vi "test Script Bitfile.vi"(8 "error in (no error)":errorcluster, 11 "TestCase in":refnum<class "Scripting API Test Case.lvclass">) -> (0 "error out":errorcluster, 3 "TestCase out":refnum<class "Scripting API Test Case.lvclass">)   [LabVIEW 2015, in "Scripting API Test Case.lvclass"]
uses:
  Scripting API Test Case.lvclass
  Scripting API/Custom Device/Engine Simulation Toolkit Custom Device Settings.ctl
  Scripting API/Bitfile/Bitfile.ctl
  Scripting API Test Case.lvclass/Scripting API Test Case.ctl
  <userlib>/_OpenG.lib/file/file.llb/Append Path to Root if Relative - Scalar__ogtk.vi
  <vilib>/addons/_JKI Toolkits/VI Tester/TestCase.llb/TestCase.lvclass
  niveristand-custom-device-testing-tools/VeriStandTestUtilities/VeriStandTestUtilities.lvlib
  Scripting API/Engine Simulation Toolkit Scripting API.lvlib
panel:
  in  "Save?":bool
  out "Output Filename":string
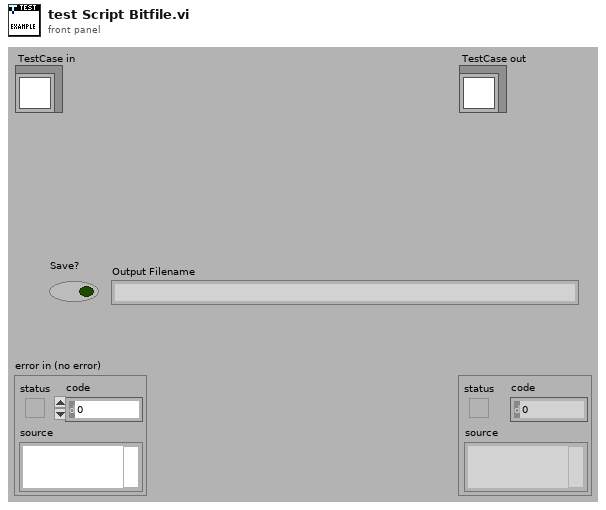
[diagram p1: front panel]
types:
  T1 = typedef "Engine Simulation Toolkit Scripting API.lvlib/Bitfile.ctl" = cluster{"RIO Device Address":string, "Bitfile Path":path}
  T2 = typedef "Engine Simulation Toolkit Scripting API.lvlib/Engine Simulation Toolkit Custom Device Settings.ctl" = cluster{"Name":string, "Execution priority":enum16{"Low", "Medium", "High"}, "Rate decimation":i32, "CPU":i32}
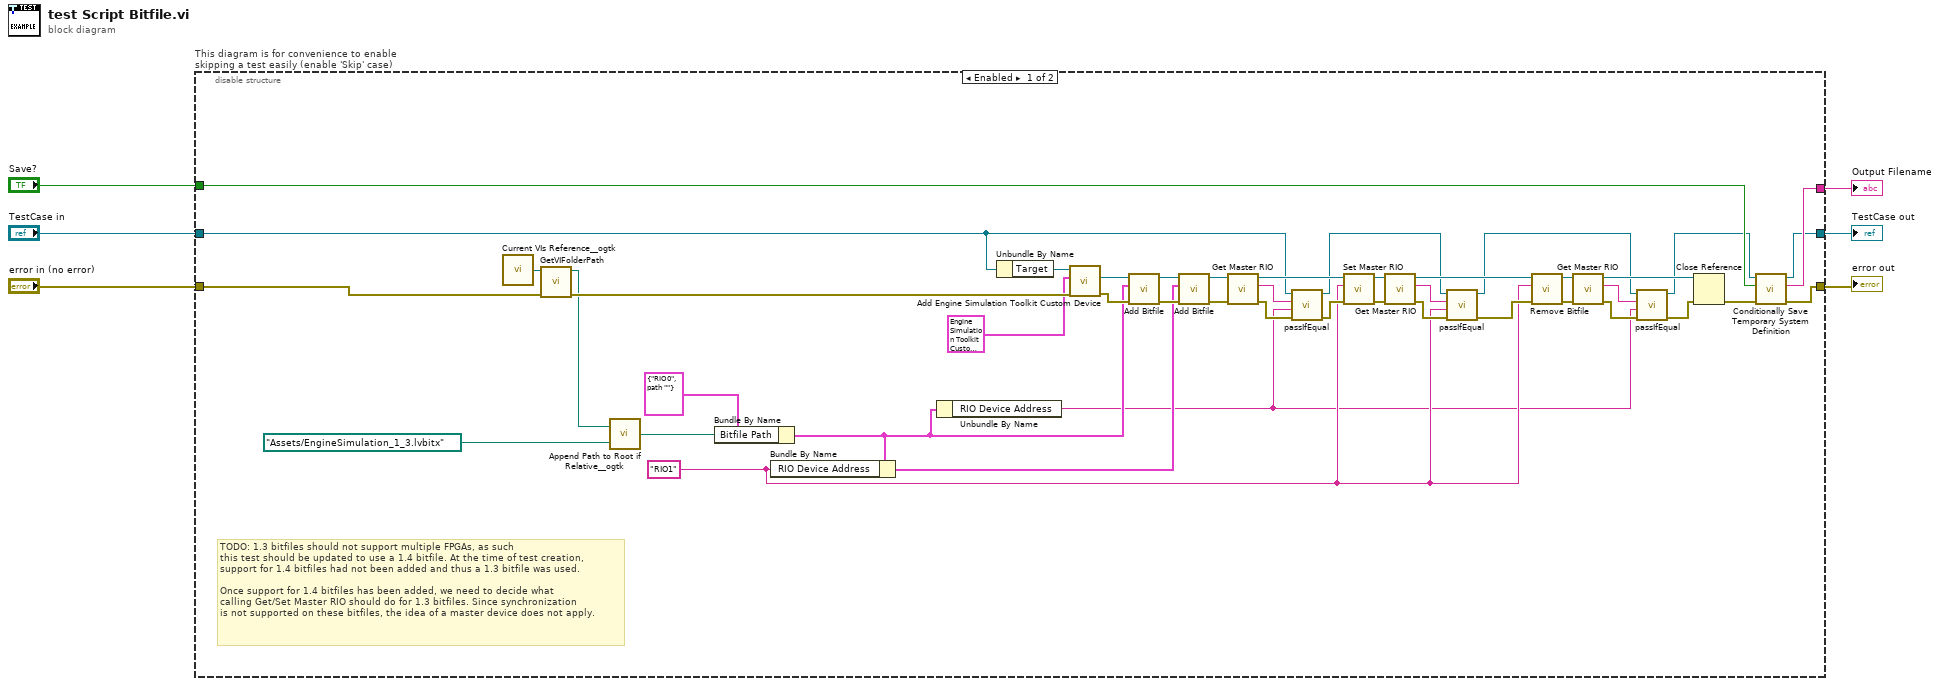
[diagram p0: block diagram]
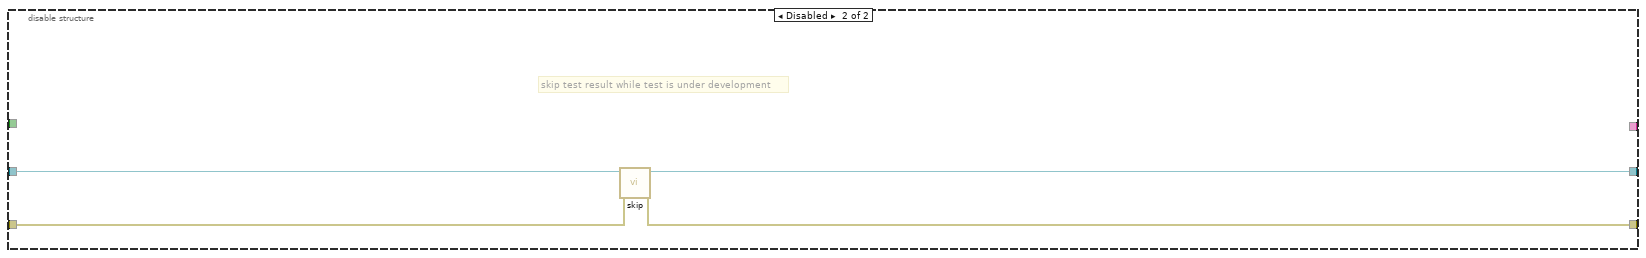
[diagram p2: hidden frame]
diagram:
  n1 = disable-structure "This diagram is for convenience to enable skipping a test easily (enable 'Skip' case)" shown="Enabled" {
    disable-tunnel: "TestCase in" -> [w10 w54]
    disable-tunnel: [w8 w52] -> w3
    disable-tunnel: [w7 w53] -> w5
    disable-tunnel: "error in (no error)" -> [w49 w51]
    disable-tunnel: [w45 _] -> w2
    disable-tunnel: "Save?" -> [w44 _]
    frame Enabled {
      w19 = "RIO1" ("RIO Device Address")
      # "TODO: 1.3 bitfiles should not support multiple FPGAs, as such\nthis test should be updated to use a 1.4 bitfile. At the time of test creation,\nsupport for 1.4 bitfiles had not been added and thus a 1.3 bitfile was used.\n\nOnce support for 1.4 bitfiles has been added, we need to decide what\ncalling Get/Set Master RIO should do for 1.3 bitfiles. Since synchronization\nis not supported on these bitfiles, the idea of a master device does not apply."
      n2 = call <userlib>:"Current VIs Reference__ogtk.vi"() -> ("Current VI's reference"=w50:refnum<vi>)  [unwired: 5 in]
      n3 = call "GetVIFolderPath.vi"("error in (no error)"=w49, "VI Reference in"=w50) -> ("error out"=w48:errorcluster, "VI Folder Path out"=w40:path)  [unwired: 8 in]
      n4 = call-poly <userlib>:"Append Path to Root if Relative__ogtk.vi"("Absolute or Relative Path"=path "Assets/EngineSimulation_1_3.lvbitx", "Root Path"=w40) -> ("Absolute or Appended Path"=w37:path)
      n5 = Bundle By Name(cluster=T1 {"RIO Device Address"="RIO0", "Bitfile Path"=path ""} ("Engine Simulation Toolkit Bitfile"), "Bitfile Path"=w37) -> (w29:T1)
      n6 = Bundle By Name(cluster=w29, "RIO Device Address"=w19) -> (w35:T1)
      n7 = Unbundle By Name(w29) -> ("RIO Device Address"=w11:string)
      n8 = Unbundle By Name(w10) -> ("Target"=w47:refnum<k24>)
      n9 = call "Add Engine Simulation Toolkit Custom Device.vi"("error in (no error)"=w48, "Settings"=T2 {"Name"="Engine Simulation Toolkit Custom Device", "Execution priority"=enum."Medium", "Rate decimation"=1, "CPU"=-2} ("Engine Simulation Toolkit Custom Device Settings"), "Target in"=w47) -> ("error out"=w41:errorcluster, "EST Custom Device"=w43:refnum<k24>)  [unwired: 6 in, 1 out]
      n10 = call "Add Bitfile.vi"("error in (no error)"=w41, "Engine Simulation Toolkit Bitfile"=w29, "EST Custom Device in"=w43) -> ("error out"=w36:errorcluster, "EST Custom Device out"=w34:refnum<k24>)  [unwired: 7 in]
      n11 = call "Add Bitfile.vi"("error in (no error)"=w36, "Engine Simulation Toolkit Bitfile"=w35, "EST Custom Device in"=w34) -> ("error out"=w33:errorcluster, "EST Custom Device out"=w32:refnum<k24>)  [unwired: 7 in]
      n12 = call "Get Master RIO.vi"("error in (no error)"=w33, "EST Custom Device in"=w32) -> ("error out"=w31:errorcluster, "RIO Device Address"=w30:string, "EST Custom Device out"=w25:refnum<k24>)  [unwired: 7 in]
      n13 = call-dynamic "passIfEqual.vi"("error in (no error)"=w31, "y"=w11, "x"=w30, "TestCase in"=w10) -> ("error out"=w28:errorcluster, "TestCase out"=w20:refnum<class "Scripting API Test Case.lvclass">)  [unwired: 6 in]
      n14 = call "Set Master RIO.vi"("error in (no error)"=w28, "RIO Device Address"=w19, "EST Custom Device in"=w25) -> ("error out"=w27:errorcluster, "EST Custom Device out"=w26:refnum<k24>)  [unwired: 7 in]
      n15 = call "Get Master RIO.vi"("error in (no error)"=w27, "EST Custom Device in"=w26) -> ("error out"=w24:errorcluster, "RIO Device Address"=w23:string, "EST Custom Device out"=w21:refnum<k24>)  [unwired: 7 in]
      n16 = call-dynamic "passIfEqual.vi"("error in (no error)"=w24, "y"=w19, "x"=w23, "TestCase in"=w20) -> ("error out"=w22:errorcluster, "TestCase out"=w12:refnum<class "Scripting API Test Case.lvclass">)  [unwired: 6 in]
      n17 = call "Remove Bitfile.vi"("error in (no error)"=w22, "RIO Device Address"=w19, "EST Custom Device in"=w21) -> ("error out"=w15:errorcluster, "EST Custom Device out"=w16:refnum<k24>)  [unwired: 7 in]
      n18 = call "Get Master RIO.vi"("error in (no error)"=w15, "EST Custom Device in"=w16) -> ("error out"=w18:errorcluster, "RIO Device Address"=w17:string, "EST Custom Device out"=w14:refnum<k24>)  [unwired: 7 in]
      n19 = call-dynamic "passIfEqual.vi"("error in (no error)"=w18, "y"=w11, "x"=w17, "TestCase in"=w12) -> ("error out"=w13:errorcluster, "TestCase out"=w9:refnum<class "Scripting API Test Case.lvclass">)  [unwired: 6 in]
      n20 = Close Reference(reference=w14, error in (no error)=w13) -> (error out=w46:errorcluster)
      n21 = call "Conditionally Save Temporary System Definition.vi"("error in (no error)"=w46, "Save?"=w44, "Test Case"=w9) -> ("error out"=w7:errorcluster, "filename"=w45:string, "Test Case"=w8:refnum<class "Scripting API Test Case.lvclass">)  [unwired: 6 in]
    }
    frame Disabled {
      # "skip test result while test is under development"
      n22 = call <vilib>:"skip.vi"("error in (no error)"=w51, "TestCase in"=w54) -> ("error out"=w53:errorcluster, "TestCase out"=w52:refnum<class "Scripting API Test Case.lvclass">)  [unwired: 8 in]
    }
  }
  "error out" <- w5
  "TestCase out" <- w3
  "Output Filename" <- w2
